vi "ShowPipetteInfo.vi"(8 "error in (no error)":errorcluster, 10 "Analysis in":refnum<class "Analysis.lvclass">, 11 "Table Control":refnum<vi>) -> (0 "error out":errorcluster)   [LabVIEW 2015]
doc: "Loads the Pipette Info from the AnalysisObject and displays the data in the Table"
uses:
  MSControl/Classes/Analysis/Analysis.lvclass
  <vilib>/Utility/miscctls.llb/LVRowAndColumnUnsignedTypeDef.ctl
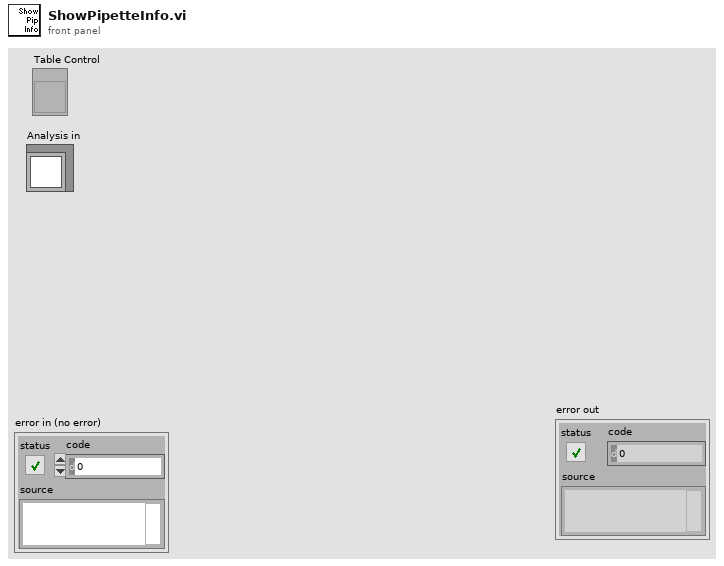
[diagram p1: front panel]
types:
  T1 = typedef "LVRowAndColumnUnsignedTypeDef.ctl" = cluster{"Row":u32, "Column":u32}
  T2 = typedef "PipetteDataArray.ctl" = string[][]
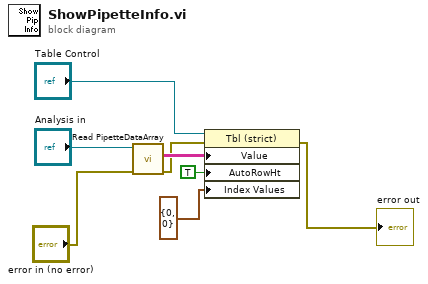
[diagram p0: block diagram]
diagram:
  n1 = call-dynamic "Read PipetteDataArray.vi"("error in (no error)"="error in (no error)", "Analysis in"="Analysis in") -> ("error out"=w3:errorcluster, "PipetteDataArray"=w5:T2)  [unwired: 7 in, 1 out]
  n2 = property class="Tbl (strict)"(reference="Table Control", error in=w3, "Value"=w5, "AutoRowHt"=TRUE ("Autosizing Row Height"), "Index Values"=T1 {"Row"=0, "Column"=0}) -> (error out=→"error out":errorcluster)  [unwired: 1 out]
